vi "HumanSwerveDrive.vi"(8 "Enable Field Oriented Drive":bool, 9 "Rotation":dbl, 10 "Y":dbl, 11 "X":dbl) -> (1 "A":dbl, 2 "Y":dbl, 3 "X":dbl)   [LabVIEW 2025]
uses:
  <vilib>/Rock Robotics/WPI/ThirdParty/JAS_Junk/TrajLib/Conv_Deg_Radians.vi
  <vilib>/Rock Robotics/WPI/ThirdParty/JAS_Junk/TrajLib/Rotation2d_CreateAngle.vi
  <vilib>/Rock Robotics/WPI/ThirdParty/JAS_Junk/TrajLib/Trajectory_Library.lvlib
panel:
  # "we switched these, hopefully it is right"
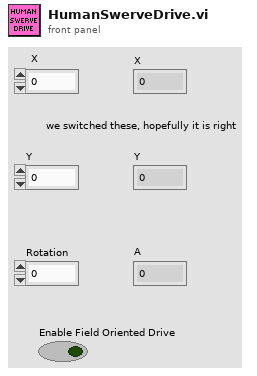
[diagram p1: front panel]
types:
  T1 = typedef "Trajectory_Library.lvlib/ROTATION2D.ctl" = cluster{"VALUE":dbl, "COS":dbl, "SIN":dbl}
  T2 = typedef "Trajectory_Library.lvlib/TRANSLATION2D.ctl" = cluster{"X":dbl, "Y":dbl}
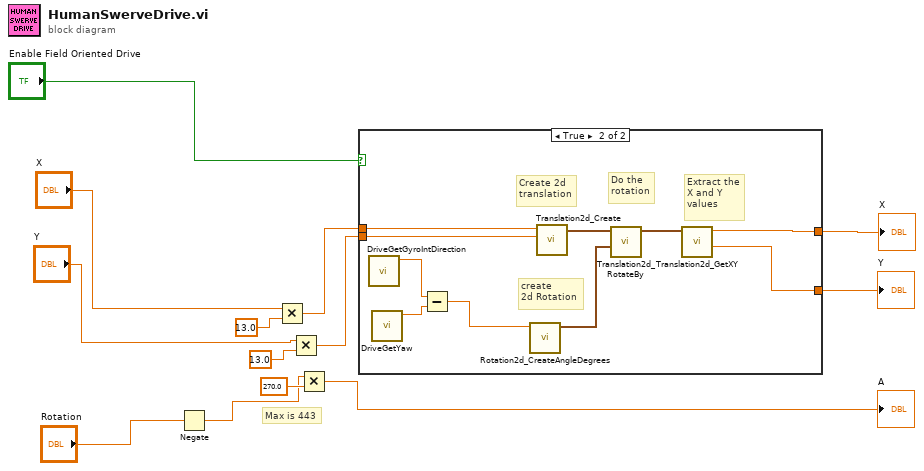
[diagram p0: block diagram]
diagram:
  # "Max is 443"
  n1 = Negate(x="Rotation") -> (-x=w1:dbl)
  n2 = Multiply(x="X", y=13.0) -> (x*y=w12:dbl)
  n3 = Multiply(x="Y", y=13.0) -> (x*y=w13:dbl)
  n4 = Multiply(x=w1, y=270.0) -> (x*y=→"A":dbl)
  n5 = case shown="True" "Enable Field Oriented Drive" {
    tunnel: w13 -> [w14 w21]
    tunnel: w12 -> [w15 w20]
    tunnel: [w15 w17] -> w5
    tunnel: [w14 w16] -> w4
    frame False {
    }
    frame True {
      # "Extract the\nX and Y \nvalues"
      # "Do the \nrotation"
      # "Create 2d\ntranslation"
      # "create\n2d Rotation"
      n6 = call "DriveGetGyroIntDirection.vi"() -> ("GyroIntDirection"=w19:dbl)  [unwired: 11 in]
      n7 = call "DriveGetYaw.vi"() -> ("Yaw"=w18:dbl)  [unwired: 11 in]
      n8 = Subtract(x=w19, y=w18) -> (x-y=w25:dbl)
      n9 = call <vilib>:"Rotation2d_CreateAngleDegrees.vi"("Angle_Degrees"=w25) -> ("ROTATION"=w23:T1)  [unwired: 10 in]
      n10 = call <vilib>:"Translation2d_Create.vi"("Y"=w21, "X"=w20) -> ("TRANSLATION"=w22:T2)  [unwired: 9 in]
      n11 = call <vilib>:"Translation2d_RotateBy.vi"("other Rotation"=w23, "In Translation"=w22) -> ("Out Translation"=w24:T2)  [unwired: 9 in]
      n12 = call <vilib>:"Translation2d_GetXY.vi"("In Translation"=w24) -> ("Y"=w16:dbl, "X"=w17:dbl)  [unwired: 9 in]
    }
  }
  "Y" <- w4
  "X" <- w5
